vi "Query Measurement Type.vi"(8 "error in (no error)":errorcluster, 11 "VISA resource name":refnum<visa-resource-name>) -> (0 "error out":errorcluster, 2 "Measurement Type":u16, 3 "VISA resource name out":refnum<visa-resource-name>)   [LabVIEW 2020, in "Agilent 34405.lvlib"]
doc: "Configures the measurement type, resolution, and range on the instrument."
uses:
  <instrlib>/Agilent 34405/Agilent 34405.lvlib
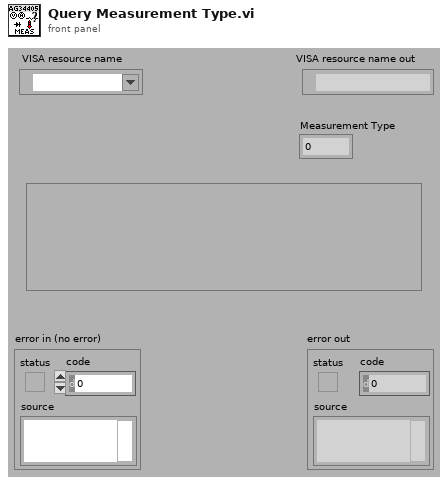
[diagram p1: front panel]
types:
  T1 = typedef "Agilent 34405.lvlib/Extended User Data.ctl" = cluster{"344XX Mode":u16, "Measurement Type":u16}
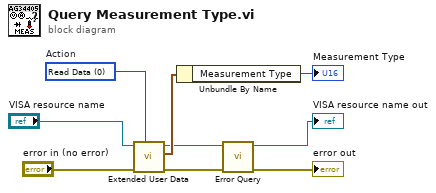
[diagram p0: block diagram]
diagram:
  w5 = 0 items=["Read Data", "Write Data", "Clear Data", "Clear ALL Data"]  # Action
  n1 = call <instrlib>:"Extended User Data.vi"("Action"=w5, "error in (no error)"="error in (no error)", "VISA resource name in"="VISA resource name") -> ("error out"=w1:errorcluster, "User Data Out"=w4:T1, "VISA resource name out"=w2:refnum<visa-resource-name>)  [unwired: 1 in, 5 out]
  n2 = Unbundle By Name(w4) -> ("Measurement Type"=→"Measurement Type":u16)
  n3 = call <instrlib>:"Error Query.vi"("error in (no error)"=w1, "VISA resource name"=w2) -> ("error out"=→"error out":errorcluster, "VISA resource name out"=→"VISA resource name out":refnum<visa-resource-name>)  [unwired: 8 out]
